vi "main_reset_panel.vi"(6 "Iteration":refnum<vi>, 7 "Runtime":refnum<vi>, 8 "Working Directory":refnum<vi>, 9 "Active Element":refnum<vi>, 10 "Simulation Log":refnum<vi>, 11 "Plant Structure":refnum<vi>) -> ()   [LabVIEW 2019]
uses:
  lib/libSimulationControl/libSimulationControl.lvlib
panel:
  # "*******************************************************************\nBiogas Plant Control\n\nAuthor: Paul Zügel\nGCSC-Frankfurt am Main 2020\n\n*******************************************************************"
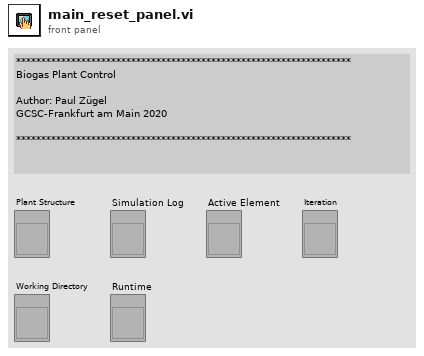
[diagram p1: front panel]
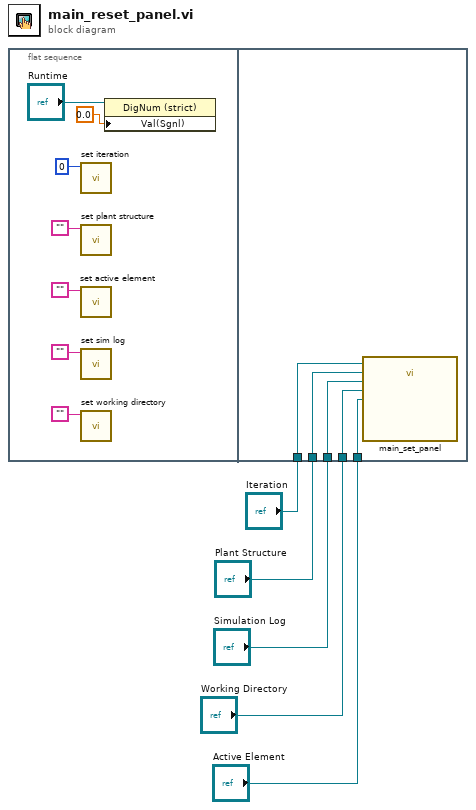
[diagram p0: block diagram]
diagram:
  n1 = flat-sequence {
    tunnel: "Plant Structure" -> [w17]
    tunnel: "Simulation Log" -> [w16]
    tunnel: "Active Element" -> [w15]
    tunnel: "Iteration" -> [w14]
    tunnel: "Working Directory" -> [w13]
    frame #0 {
      n2 = call "set iteration.vi"("iter"=0 ("Value")) -> ()  [unwired: 10 in, 1 out]
      n3 = call "set plant structure.vi"("structure"="") -> ()  [unwired: 10 in, 1 out]
      n4 = call "set active element.vi"("elem"="") -> ()  [unwired: 10 in, 1 out]
      n5 = call "set sim log.vi"("log"="") -> ()  [unwired: 10 in, 1 out]
      n6 = call "set working directory.vi"("dir"="") -> ()  [unwired: 10 in, 1 out]
      n7 = property on="Property Node" class="DigNum (strict)"(reference="Runtime", "Val(Sgnl)"=0.0 ("Value (Signaling)")) -> ()  [unwired: 1 in, 2 out]
    }
    frame #1 {
      n8 = call "main_set_panel.vi"("Active Element"=w15, "Working Directory"=w13, "Simulation Log"=w16, "Plant Structure"=w17, "Iteration"=w14) -> ()  [unwired: 7 in]
    }
  }
